vi "3ALABVIEW (1).vi"() -> ()   [LabVIEW 2013]
panel:
  in  "x":i32
  out "Array":i32[](array[numeric])
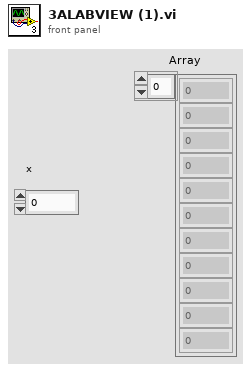
[diagram p1: front panel]
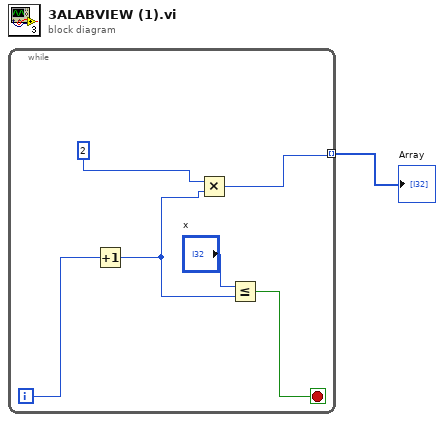
[diagram p0: block diagram]
diagram:
  n1 = while {
    tunnel: [w4] -> w1 mode=indexing
    i -> [w7]
    stop <- w6 stop-if-true
    n2 = Increment(x=w7) -> (x+1=w3:i32)
    n3 = Multiply(x=2 ("x+1"), y=w3) -> (x*y=w4:i32)
    n4 = Less Or Equal?(x="x", y=w3) -> (x <= y?=w6:bool)
  }
  "Array" <- w1
